vi "Compile Device Settings.vi"(8 "error in (no error)":errorcluster, 11 "Device Ref in":T1 format="%.0x") -> (0 "error out":errorcluster, 2 "Device Settings":T2, 3 "Device Ref out":T1 format="%.0x")   [LabVIEW 2014, in "SLSC configuration System Explorer.lvlib"]
uses:
  SLSC configuration System Explorer.lvlib
  Shared/Type Defs/Device Settings.ctl
  <vilib>/NI Veristand/Custom Device API/Custom Device Item Ref.ctl
  Shared/Constants.vi
  <vilib>/NI Veristand/Custom Device API/Get Item Property (U16).vi
  <vilib>/NI Veristand/Custom Device API/Get Item Property (U32).vi
  <vilib>/NI Veristand/Custom Device API/Get Item Property (Dependent File).vi
  <vilib>/NI Veristand/Custom Device API/Get Item Property (String).vi
  <vilib>/NI Veristand/Custom Device API/Custom Device API.lvlib
  Shared/SLSC configuration Shared.lvlib
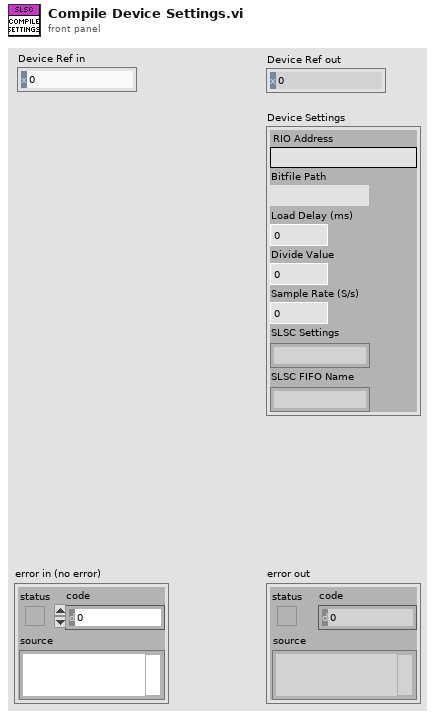
[diagram p1: front panel]
types:
  T1 = typedef "Custom Device API.lvlib/Custom Device Item Ref.ctl" = u64
  T2 = typedef "SLSC configuration Shared.lvlib/Device Settings.ctl" = cluster{"RIO Address":string, "Bitfile Path":path, "Load Delay (ms)":u32, "Divide Value":u8, "Sample Rate (S/s)":u32, "SLSC Settings":string, "SLSC FIFO Name":string}
  T3 = typedef "Custom Device API.lvlib/Custom Device Target Type.ctl" = enum16{"PharLap", "VxWorks", "Windows"}
  T4 = typedef "Custom Device API.lvlib/Dependent File Optional Info.ctl" = cluster{"Version":string, "RTDestination":path, "ForceDownload":bool, "SupportedTarget":string, "MD5":string}
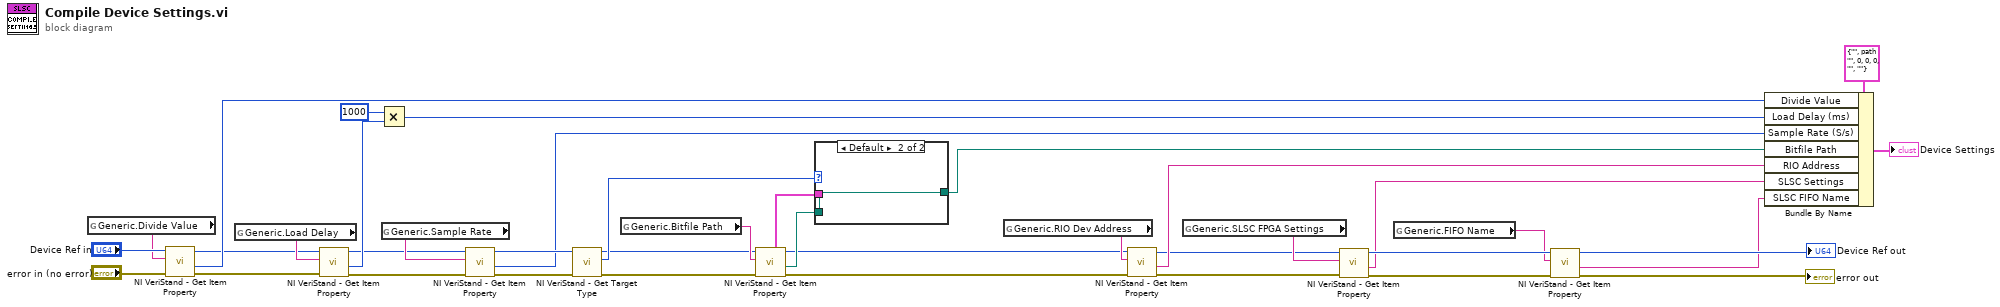
[diagram p0: block diagram]
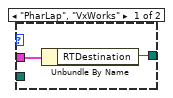
[diagram p2: hidden frame]
diagram:
  n1 = global read "Constants.vi" "Generic.Divide Value"() -> (w25:string)
  n2 = call-poly <vilib>:"NI VeriStand - Get Item Property.vi"("error in (no error)"="error in (no error)", "Property Name"=w25, "Item Ref in"="Device Ref in") -> ("error out"=w15:errorcluster, "Value"=w27:u16, "Item Ref out"=w16:T1)  [unwired: 5 in, 1 out]
  n3 = global read "Constants.vi" "Generic.Load Delay"() -> (w17:string)
  n4 = call-poly <vilib>:"NI VeriStand - Get Item Property.vi"("error in (no error)"=w15, "Property Name"=w17, "Item Ref in"=w16) -> ("error out"=w18:errorcluster, "Value"=w28:u16, "Item Ref out"=w19:T1)  [unwired: 5 in, 1 out]
  n5 = Multiply(x=u32 1000, y=w28) -> (x*y=w30:u32)
  n6 = global read "Constants.vi" "Generic.Sample Rate"() -> (w20:string)
  n7 = call-poly <vilib>:"NI VeriStand - Get Item Property.vi"("error in (no error)"=w18, "Property Name"=w20, "Item Ref in"=w19) -> ("error out"=w32:errorcluster, "Value"=w31:u32, "Item Ref out"=w33:T1)  [unwired: 5 in, 1 out]
  n8 = call <vilib>:"NI VeriStand - Get Target Type.vi"("error in (no error)"=w32, "Item Ref in"=w33) -> ("error out"=w34:errorcluster, "Target Type"=w35:T3, "Item Ref out"=w13:T1)  [unwired: 7 in]
  n9 = global read "Constants.vi" "Generic.Bitfile Path"() -> (w21:string)
  n10 = call-poly <vilib>:"NI VeriStand - Get Item Property.vi"("error in (no error)"=w34, "Property Name"=w21, "Item Ref in"=w13) -> ("error out"=w22:errorcluster, "Path"=w36:path, "Item Ref out"=w23:T1, "OptionalInfo"=w38:T4)  [unwired: 4 in, 1 out]
  n11 = case shown="Default" w35 {
    tunnel: [w40 w42] -> w37
    tunnel: w36 -> [_ w42]
    tunnel: w38 -> [w41 _]
    frame "PharLap", "VxWorks" {
      n12 = Unbundle By Name(w41) -> ("RTDestination"=w40:path)
    }
    frame Default {
    }
  }
  n13 = global read "Constants.vi" "Generic.RIO Dev Address"() -> (w24:string)
  n14 = call-poly <vilib>:"NI VeriStand - Get Item Property.vi"("error in (no error)"=w22, "Property Name"=w24, "Item Ref in"=w23) -> ("error out"=w9:errorcluster, "Value"=w26:string, "Item Ref out"=w8:T1)  [unwired: 5 in, 1 out]
  n15 = global read "Constants.vi" "Generic.SLSC FPGA Settings"() -> (w10:string)
  n16 = call-poly <vilib>:"NI VeriStand - Get Item Property.vi"("error in (no error)"=w9, "Property Name"=w10, "Item Ref in"=w8) -> ("error out"=w7:errorcluster, "Value"=w2:string, "Item Ref out"=w6:T1)  [unwired: 5 in, 1 out]
  n17 = global read "Constants.vi" "Generic.FIFO Name"() -> (w5:string)
  n18 = call-poly <vilib>:"NI VeriStand - Get Item Property.vi"("error in (no error)"=w7, "Property Name"=w5, "Item Ref in"=w6) -> ("error out"=→"error out":errorcluster, "Value"=w1:string, "Item Ref out"=→"Device Ref out":T1)  [unwired: 5 in, 1 out]
  n19 = Bundle By Name(cluster=T2 {"RIO Address"="", "Bitfile Path"=path "", "Load Delay (ms)"=0, "Divide Value"=0, "Sample Rate (S/s)"=0, "SLSC Settings"="", "SLSC FIFO Name"=""}, "Divide Value"=w27, "Load Delay (ms)"=w30, "Sample Rate (S/s)"=w31, "Bitfile Path"=w37, "RIO Address"=w26, "SLSC Settings"=w2, "SLSC FIFO Name"=w1) -> (→"Device Settings":T2)
